vi "Convert TDMS Log Files to ASCII.vi"() -> ()   [LabVIEW 2010, in "TDMS to ASCII Convert.lvlib"]
uses:
  TDMS to ASCII Convert.lvlib
  Stop FGV Commands.ctl
  Global.vi
panel:
  in  "Destination directory":path
  in  "Recursive?":bool=TRUE
  in  "Directory of TDMS files":path
  out "Progress":u8(slide) scale=0.0..100.0
  in  "Abort":bool
  in  "Start":bool
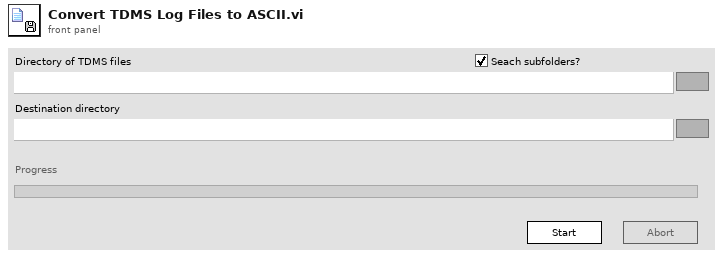
[diagram p1: front panel]
types:
  T1 = typedef "TDMS to ASCII Convert.lvlib/Stop FGV Commands.ctl" = enum16{"Write", "Read", "Reset"}
  T2 = enum8{"Enabled", "Disabled", "Disabled and Grayed Out"}
  T3 = enum32{"invalid app kind", "Development System", "Run Time System", "Student Edition", "Embedded LabVIEW", "Evaluation", "Custom"}
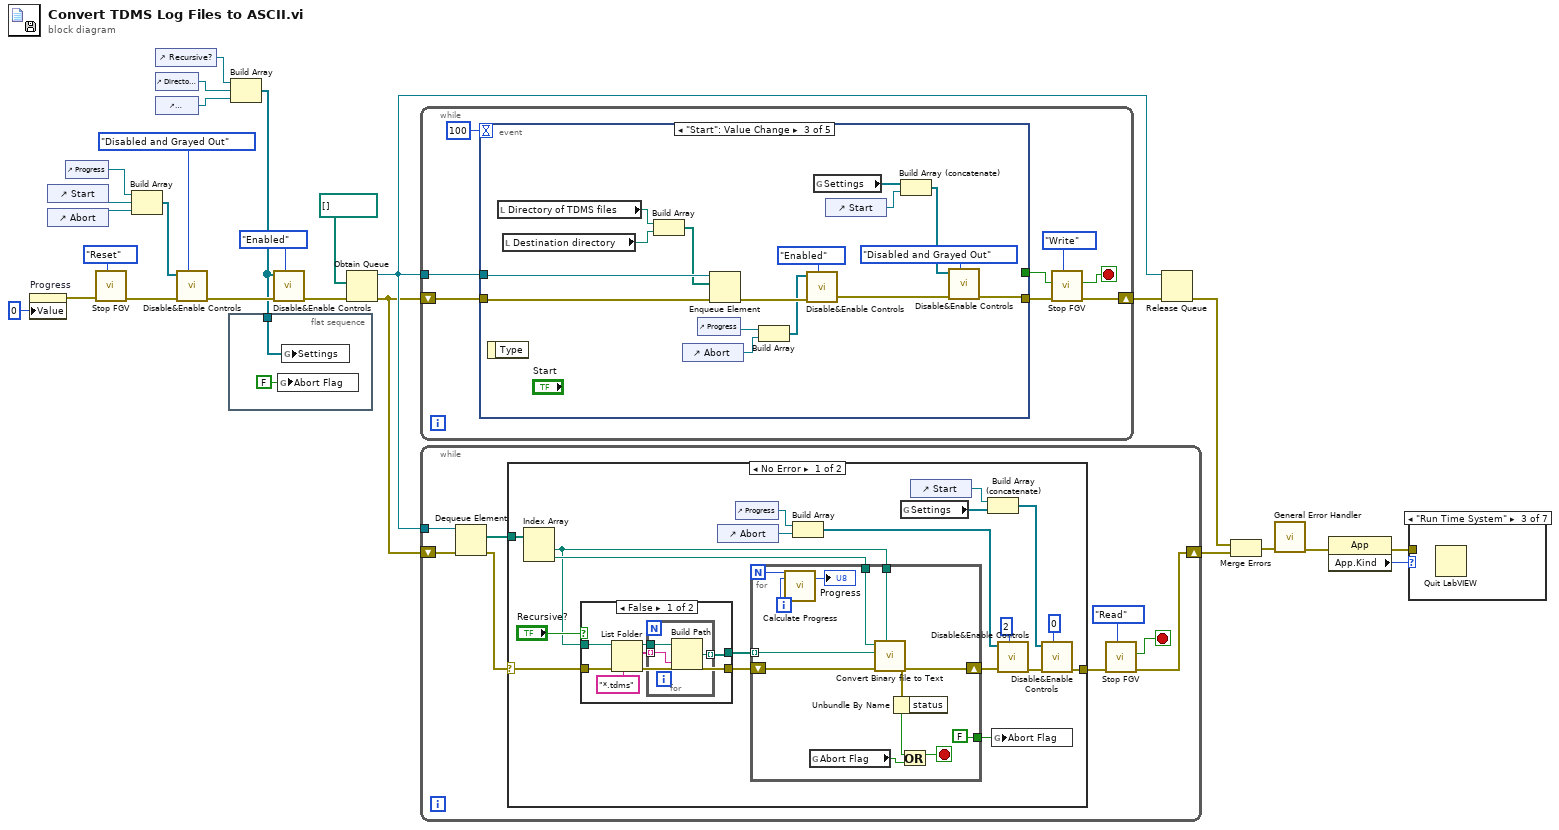
[diagram p0: block diagram]
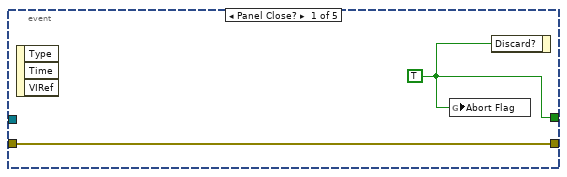
[diagram p8: hidden frame]
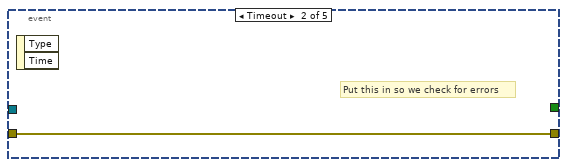
[diagram p9: hidden frame]
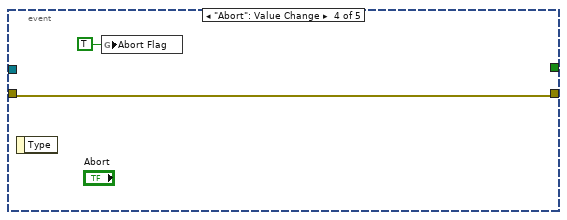
[diagram p10: hidden frame]
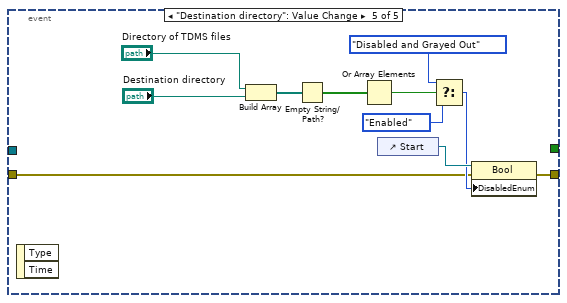
[diagram p11: hidden frame]
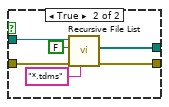
[diagram p12: hidden frame]
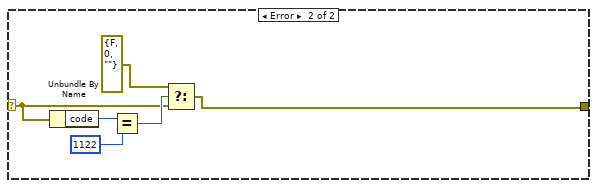
[diagram p13: hidden frame]
diagram:
  n1 = property on="Progress" class="Slide (strict)"("Value"=u8 0 ("Progress")) -> (error out=w7:errorcluster)  [unwired: 2 in, 1 out]
  n2 = control-ref of="Start"() -> (w20:refnum<vi>)
  n3 = control-ref of="Abort"() -> (w19:refnum<vi>)
  n4 = control-ref of="Progress"() -> (w21:refnum<vi>)
  n5 = call "Stop FGV.vi"("Command"=Stop_FGV_Commands."Reset", "error in (no error)"=w7) -> ("error out"=w3:errorcluster)  [unwired: 7 in, 2 out]
  n6 = Build Array(w21, w20, w19) -> (w18:refnum<vi>[])
  n7 = control-ref of="Recursive?"() -> (w24:refnum<vi>)
  n8 = control-ref of="Directory of TDMS files"() -> (w25:refnum<vi>)
  n9 = control-ref of="Destination directory"() -> (w26:refnum<vi>)
  n10 = call "Disable&Enable Controls.vi"("State"=T2."Disabled and Grayed Out", "error in (no error)"=w3, "Controls"=w18) -> ("error out"=w22:errorcluster)  [unwired: 8 in]
  n11 = flat-sequence {
    tunnel: w2 -> [w27]
    frame #0 {
      n12 = global write "Global.vi" "Abort Flag"(FALSE) -> ()
      n13 = global write "Global.vi" "Settings"(w27) -> ()
    }
  }
  n14 = Build Array(w24, w25, w26) -> (w2:refnum<vi>[])
  n15 = call "Disable&Enable Controls.vi"("State"=T2."Enabled" ("Disabled"), "error in (no error)"=w22, "Controls"=w2) -> ("error out"=w16:errorcluster)  [unwired: 8 in]
  n16 = Obtain Queue(element data type=path[] [], error in (no error)=w16) -> (queue out=w12:refnum<queue>, error out=w11:errorcluster)  [unwired: 3 in, 1 out]
  n17 = while {
    shift-right: [w33] -> w14
    shift-left: w11 -> [w36]
    tunnel: w12 -> [w35]
    stop <- w32 stop-if-true
    n18 = event shown="[2] \"Start\": Value Change" {
      selector: _ -> [_ _ _ _ _]
      dyn-events: _ -> [_ _ _ _ _]
      timeout: 100 -> [_ _ _ _ _]
      tunnel: [w37 _ _ _ _] -> w30
      tunnel: w36 -> [w38 w39 w55 w56 w58]
      tunnel: [w38 w39 w47 w56 w62] -> w34
      tunnel: w35 -> [_ _ w54 _ _]
      event Panel Close? {
        w37 = TRUE
        n19 = event-data() -> ()  [unwired: 1 in, 3 out]
        n20 = global write "Global.vi" "Abort Flag"(w37) -> ()
        n21 = event-data("Discard?"=w37) -> ()  [unwired: 1 in, 1 out]
      }
      event Timeout {
        # "Put this in so we check for errors"
        n22 = event-data() -> ()  [unwired: 1 in, 2 out]
      }
      event "Start": Value Change {
        n23 = event-data() -> ()  [unwired: 1 in, 1 out]
        n24 = local read "Directory of TDMS files"() -> (w53:path)
        n25 = local read "Destination directory"() -> (w40:path)
        n26 = Build Array(w53, w40) -> (w52:path[])
        n27 = control-ref of="Abort"() -> (w46:refnum<vi>)
        n28 = control-ref of="Progress"() -> (w45:refnum<vi>)
        n29 = Enqueue Element(queue=w54, element=w52, error in (no error)=w55) -> (error out=w51:errorcluster)  [unwired: 1 in, 2 out]
        n30 = Build Array(w45, w46) -> (w44:refnum<vi>[])
        n31 = call "Disable&Enable Controls.vi"("State"=T2."Enabled", "error in (no error)"=w51, "Controls"=w44) -> ("error out"=w49:errorcluster)  [unwired: 8 in]
        n32 = global read "Global.vi" "Settings"() -> (w41:refnum<vi>[])
        n33 = control-ref of="Start"() -> (w43:refnum<vi>)
        n34 = Build Array (concatenate)(w41, w43) -> (w42:refnum<vi>[])
        n35 = call "Disable&Enable Controls.vi"("State"=T2."Disabled and Grayed Out", "error in (no error)"=w49, "Controls"=w42) -> ("error out"=w47:errorcluster)  [unwired: 8 in]
      }
      event "Abort": Value Change {
        n36 = event-data() -> ()  [unwired: 1 in, 1 out]
        n37 = global write "Global.vi" "Abort Flag"(TRUE ("Abort Flag")) -> ()
      }
      event "Destination directory": Value Change {
        n38 = event-data() -> ()  [unwired: 1 in, 2 out]
        n39 = Build Array("Directory of TDMS files", "Destination directory") -> (w66:path[])
        n40 = Empty String/Path?(string/path=w66) -> (empty?=w59:bool[])
        n41 = Or Array Elements(Boolean array=w59) -> (logical OR=w65:bool)
        n42 = control-ref of="Start"() -> (w61:refnum<vi>)
        n43 = Select(t=T2."Disabled and Grayed Out" ("State"), s=w65, f=T2."Enabled") -> (s? t:f=w60:T2)
        n44 = property class="Bool"(reference=w61, error in=w58, "DisabledEnum"=w60) -> (error out=w62:errorcluster)  [unwired: 1 out]
      }
    }
    n45 = call "Stop FGV.vi"("Command"=Stop_FGV_Commands."Write", "error in (no error)"=w34, "Stop?"=w30) -> ("error out"=w33:errorcluster, "Latched Stop"=w32:bool)  [unwired: 6 in, 1 out]
  }
  n46 = while {
    shift-right: [w73] -> w9
    shift-left: w11 -> [w76]
    tunnel: w12 -> [w75]
    stop <- w72 stop-if-true
    n47 = Dequeue Element(queue=w75, error in (no error)=w76) -> (element=w70:path[], error out=w74:errorcluster)  [unwired: 1 in, 2 out]
    n48 = case shown="No Error" w74 {
      selector: w74 -> [w77 w126]
      tunnel: [w90 w125] -> w69
      tunnel: w70 -> [w86 _]
      frame No Error {
        n49 = Index Array(array=w86) -> (element #1=w78:path, element #2=w80:path)  [unwired: 2 in]
        n50 = case shown="False" "Recursive?" {
          tunnel: w78 -> [w113 w123]
          tunnel: w77 -> [w114 w120]
          tunnel: [w110 w119] -> w84
          tunnel: [w108 w118] -> w83
          frame False {
            n51 = List Folder(path=w113, pattern="*.tdms", error in=w114) -> (path out=w112:path, filenames=w111:string[], error out=w110:errorcluster)  [unwired: 1 in, 1 out]
            n52 = for {
              tunnel: w112 -> [w117]
              tunnel: w111 -> [w116] mode=indexing
              tunnel: [w115] -> w108 mode=indexing
              n53 = Build Path(base path=w117, name or relative path=w116) -> (appended path=w115:path)
            }
          }
          frame True {
            n54 = call <vilib>:"Recursive File List.vi"("pattern"="*.tdms", "error in (no error)"=w120, "Treat LLBs as Folders?"=FALSE, "Folder Path"=w123) -> ("error out"=w119:errorcluster, "All Files in Dir"=w118:path[])  [unwired: 3 in, 3 out]
          }
        }
        n55 = control-ref of="Abort"() -> (w93:refnum<vi>)
        n56 = control-ref of="Progress"() -> (w94:refnum<vi>)
        n57 = for {
          N -> [w105]
          tunnel: w83 -> [w99] mode=indexing
          shift-right: [w96] -> w82
          shift-left: w84 -> [w102]
          tunnel: [FALSE] -> w81
          tunnel: w80 -> [w101]
          tunnel: w78 -> [w100]
          i -> [w106]
          stop <- w98 stop-if-true
          n58 = call "Calculate Progress.vi"("Total Iterations"=w105, "Current Iteration"=w106) -> ("Progress"=→"Progress":u8)  [unwired: 17 in]
          n59 = global read "Global.vi" "Abort Flag"() -> (w103:bool)
          n60 = call "Convert Binary file to Text.vi"("Originating directory"=w100, "error in (no error)"=w102, "TDMS File Path"=w99, "Destination directory"=w101) -> ("error out"=w96:errorcluster)  [unwired: 7 in]
          n61 = Unbundle By Name(w96) -> ("status"=w97:bool)
          n62 = Or(x=w97, y=w103) -> (x .or. y?=w98:bool)
        }
        n63 = Build Array(w94, w93) -> (w92:refnum<vi>[])
        n64 = global read "Global.vi" "Settings"() -> (w79:refnum<vi>[])
        n65 = control-ref of="Start"() -> (w88:refnum<vi>)
        n66 = Build Array (concatenate)(w88, w79) -> (w87:refnum<vi>[])
        n67 = global write "Global.vi" "Abort Flag"(w81) -> ()
        n68 = call "Disable&Enable Controls.vi"("State"=2, "error in (no error)"=w82, "Controls"=w92) -> ("error out"=w91:errorcluster)  [unwired: 8 in]
        n69 = call "Disable&Enable Controls.vi"("State"=0, "error in (no error)"=w91, "Controls"=w87) -> ("error out"=w90:errorcluster)  [unwired: 8 in]
      }
      frame Error {
        n70 = Unbundle By Name(w126) -> ("code"=w129:i32)
        n71 = Equal?(x=w129, y=1122) -> (x = y?=w127:bool)
        n72 = Select(t=errorcluster {"status"=FALSE, "code"=0, "source"=""}, s=w127, f=w126) -> (s? t:f=w125:errorcluster)
      }
    }
    n73 = call "Stop FGV.vi"("Command"=Stop_FGV_Commands."Read", "error in (no error)"=w69) -> ("error out"=w73:errorcluster, "Latched Stop"=w72:bool)  [unwired: 7 in, 1 out]
  }
  n74 = Release Queue(queue=w12, error in (no error)=w14) -> (error out=w13:errorcluster)  [unwired: 1 in, 2 out]
  n75 = Merge Errors(w13, w9) -> (w8:errorcluster)
  n76 = call <vilib>:"General Error Handler.vi"("error in (no error)"=w8) -> ("error out"=w5:errorcluster)  [unwired: 10 in, 4 out]
  n77 = property class="App"(error in=w5) -> (error out=w1:errorcluster, "App.Kind"=w4:T3)  [unwired: 1 in, 1 out]
  n78 = case shown="\"Run Time System\"" w4 {
    tunnel: w1 -> [_ _ _ _ _ _ _]
    frame "invalid app kind", Default {
    }
    frame "Development System" {
    }
    frame "Run Time System" {
      n79 = Quit LabVIEW() -> ()  [unwired: 1 in]
    }
    frame "Student Edition" {
    }
    frame "Embedded LabVIEW" {
    }
    frame "Evaluation" {
    }
    frame "Custom" {
    }
  }
